vi "Receiver_Example - 2 Channel - Experiment.vi"() -> ()   [LabVIEW 2022 SP3]
panel:
  out "Iterations 2":i32
  in  "OFDM - 4QAM/16QAM":bool
  out "Error out 2":errorcluster
  in  "Tab Control 2":enum32{"OFDM - 4QAM", "16QAM"}(tab)
  in  "Tab Control":enum32{"USRP Parameters", "Rx Info", "BER"}(tab)
  in  "USRP ControledParameters":T1={"Active Antenna"="RX2", "Gain (dB)"=10.0, "Carrier Frequency"=2400000000.0, "IQ Rate"=2000000.0, "Active channels"="0"} {"IQ Rate" format="%#_6p"; "Carrier Frequency" format="%#_6p"; "Gain (dB)" format="%#_6f"}
  in  "Device selection":refnum<k15>="RIO0"
  in  "Trigger level":dbl=0.005 format="%f"
  out "?":T2
  out "SIG valid?":bool
  out "Frequency offset":dbl
  out "Coerced Parameters":T3={"IQ Rate"=100000.0, "Carrier  Freq."=100000.0, "Gain"=0.0} {"Gain" format="%#_6f"; "Carrier  Freq." format="%#_6p"; "IQ Rate" format="%#_6p"}
  out "Error out":errorcluster
  in  "Boolean":bool
  in  "Expected message LP":string="Non Critical Data\nNon Critical Data\nNon Critical Data\nNon Critical Data\nNon Critical Data"
  in  "Record BER":bool
  in  "Refresh Button":bool
  out "Inst. BER LP":dbl format="%#_4g"
  out "No. Bits LP":dbl
  out "Acum. Err LP":dbl
  out "Acc. BER LP":dbl format="%#_4g"
  in  "Expected message 2 HP":string="Critical Dataaaaa\nCritical Dataaaaa\nCritical Dataaaaa\nCritical Dataaaaa\nCritical Dataaaaa"
  out "Inst. BER HP":dbl format="%#_4g"
  out "Acum. Err HP":dbl
  out "No. Bits HP":dbl
  out "Acc. BER  HP":dbl format="%#_4g"
  out "Expected message LP Detected":string="Non Critical Data\nNon Critical Data\nNon Critical Data\nNon Critical Data\nNon Critical Data"
  out "Expected message  HP  Detected":string="Critical Dataaaaa\nCritical Dataaaaa\nCritical Dataaaaa\nCritical Dataaaaa\nCritical Dataaaaa"
  in  "Boolean 2":bool
  out "Constellation Map":cdb[](graph)
  out "Low-Power Decoded Message":string
  out "High-Power Decoded Message":string
  out "Low-Power BER Graph":dbl(graph)
  out "High-Power BER Graph":dbl(graph)
  out "Low-Power Instantaneous BER Graph":u8(slide) scale=0.0..100.0
  out "High-Power Instantaneous BER Graph":u8(slide) scale=0.0..100.0
  in  "Low-Power Window Size":dbl=15.0 format="%#_6p"
  in  "High-Power Window Size":dbl=15.0 format="%#_6p"
  out "Reconstructed Image":T4(plugin-control)
  out "Expected message  HP  Detected 2":string="Critical Dataaaaa\nCritical Dataaaaa\nCritical Dataaaaa\nCritical Dataaaaa\nCritical Dataaaaa"
  in  "Boolean 3":bool
  in  "High-Power Window Size 2":dbl=15.0 format="%#_6p"
  out "High-Power Instantaneous BER Graph 2":u8(slide) scale=0.0..100.0
  out "High-Power BER Graph 2":dbl(graph)
  out "No. Bits HP 2":dbl
  out "Acc. BER  HP 2":dbl format="%#_4g"
  out "Acum. Err HP 2":dbl
  out "Inst. BER HP 2":dbl format="%#_4g"
  in  "Expected message 2 HP 2":string="Critical Dataaaaa\nCritical Dataaaaa\nCritical Dataaaaa\nCritical Dataaaaa\nCritical Dataaaaa"
  out "High-Power Decoded Message 2":string
  in  "Record BER 2":bool
  out "Constellation Map 2":cdb[](graph)
  out "Frequency offset 2":dbl
  out "SIG valid? 2":bool
  in  "Refresh Button 2":bool
  out "Reconstructed Image":T4(plugin-control)
  out "Iterations":i32
  in  "error in (no error)":errorcluster
  # "OFDM Superposition Coded Receiver"
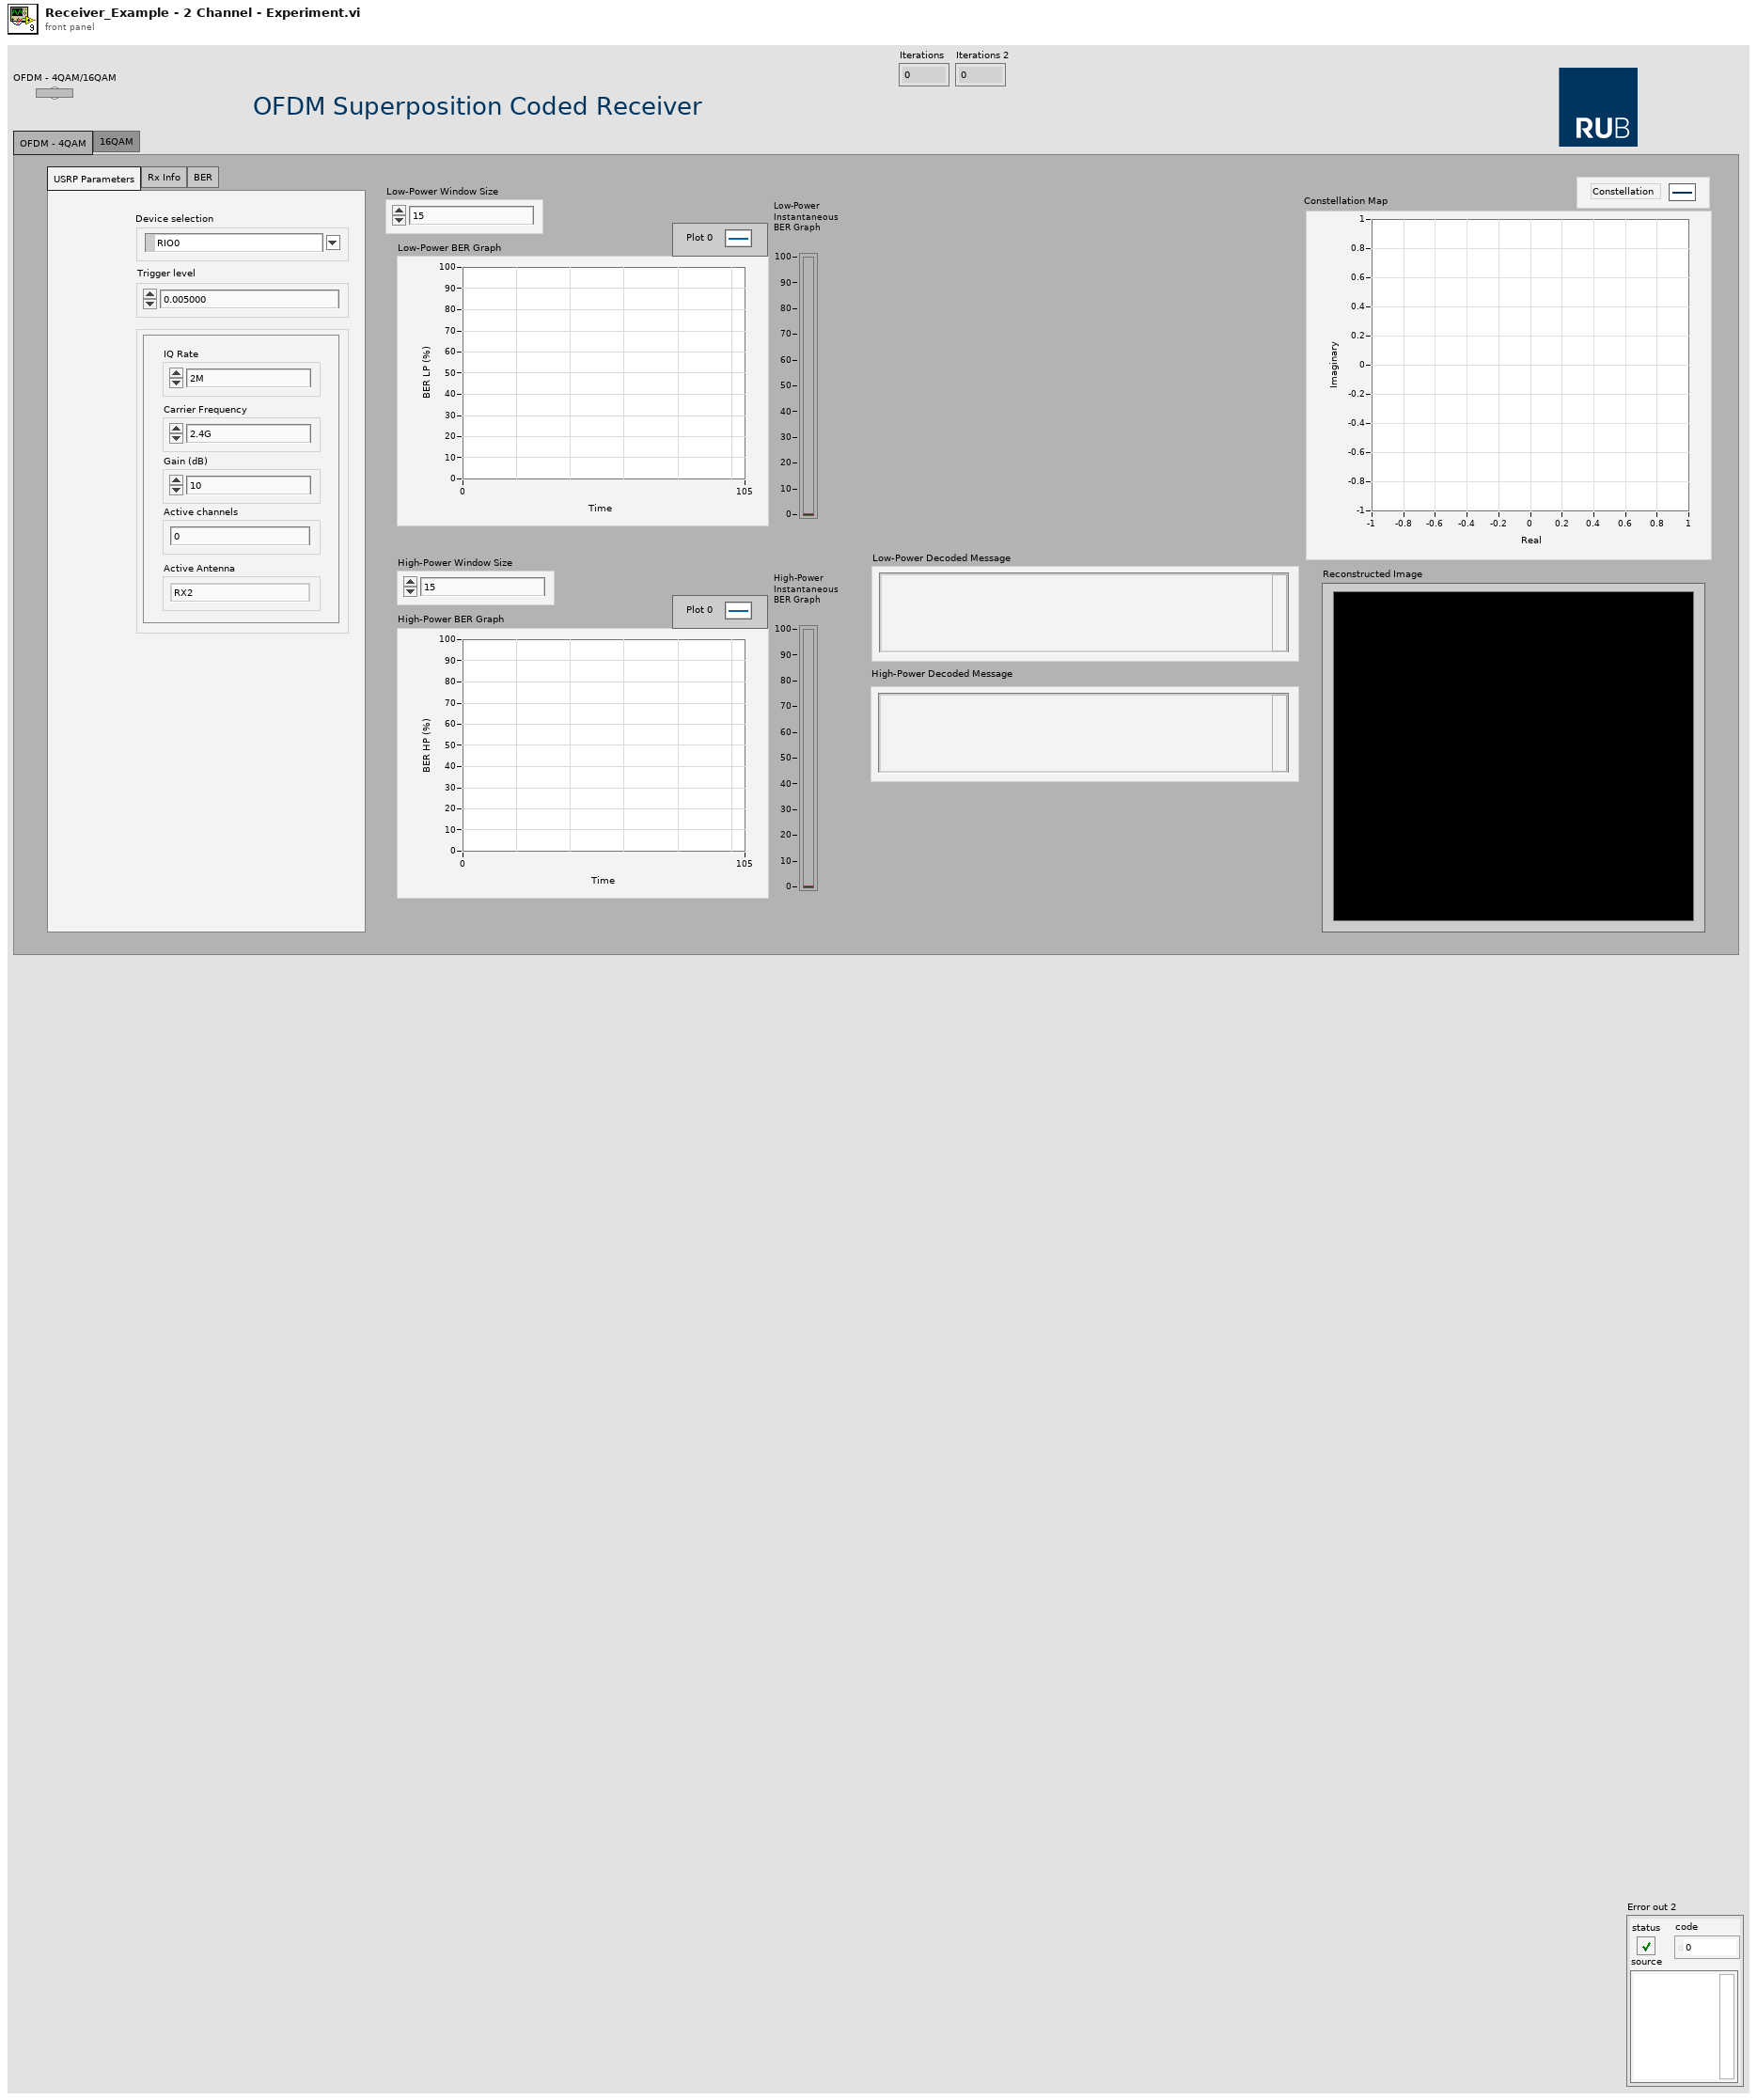
[diagram p1: front panel]
types:
  T1 = cluster{"Active Antenna":string, "Gain (dB)":dbl, "Carrier Frequency":dbl, "IQ Rate":dbl, "Active channels":string}
  T2 = cluster{"Modulation type":enum16{"QPSK(4QAM)", "64QAM", "16QAM", "BPSK"}, "BCC rate (k/n)":enum16{"1/2", "2/3", "3/4"}}
  T3 = cluster{"IQ Rate":dbl, "Carrier  Freq.":dbl, "Gain":dbl}
  T4 = typedef "IMAQ Image.ctl" = refnum<image>
  T5 = cluster{"coerced IQ rate":dbl, "coerced carrier frequency":dbl, "coerced gain":dbl}
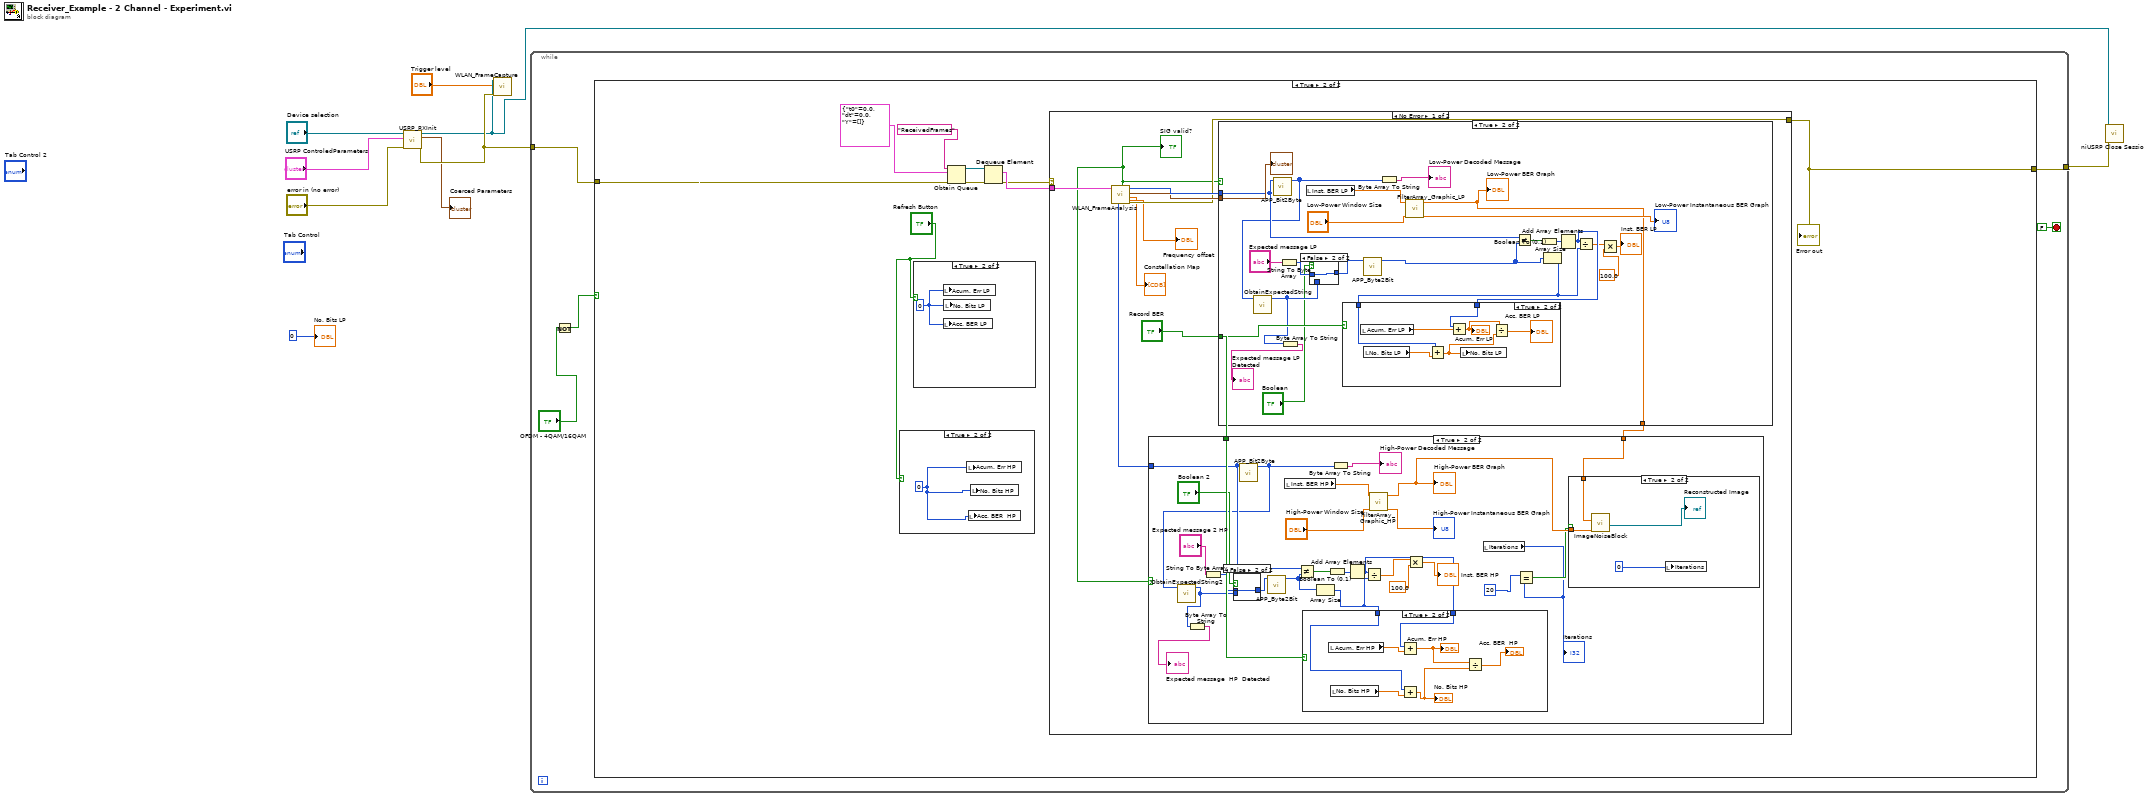
[diagram p0: block diagram]
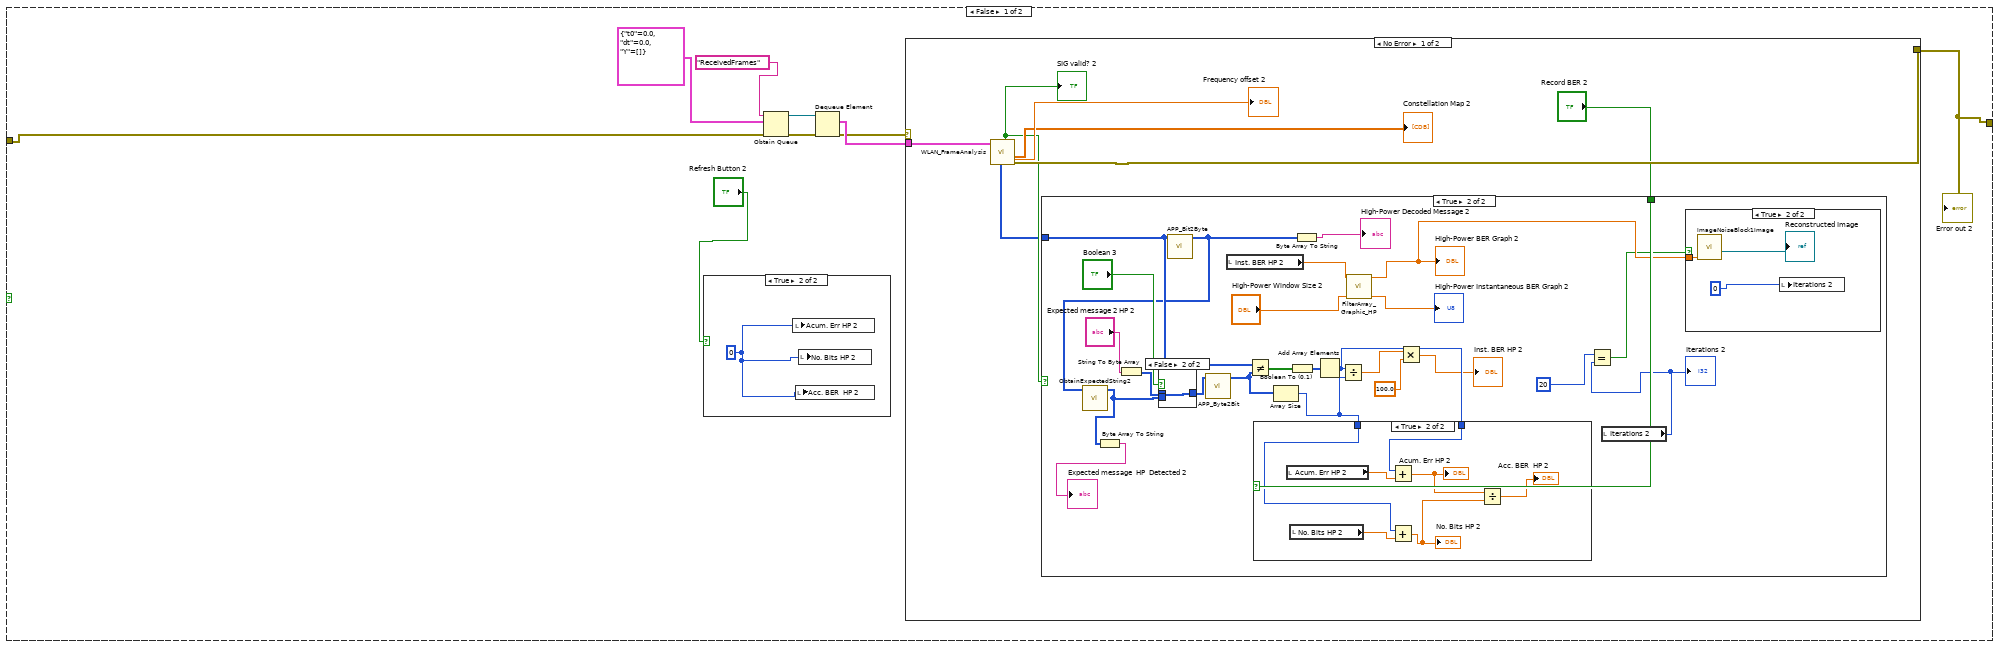
[diagram p2: hidden frame]
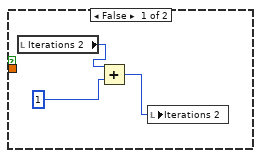
[diagram p5: hidden frame]
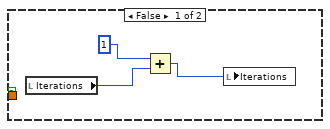
[diagram p13: hidden frame]
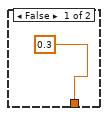
[diagram p15: hidden frame]
diagram:
  n1 = call "USRP_RXInit.vi"("device names"="Device selection", "USRP ControledParameters"="USRP ControledParameters", "error in (no error)"="error in (no error)") -> ("session handle out"=w6:refnum<k15>, "USRP CoercedParamters"=→"Coerced Parameters":T5, "error out"=w8:errorcluster)  [unwired: 5 in]
  n2 = call "WLAN_FrameCapture.vi"("error in (no error)"=w8, "Trigger level"="Trigger level", "session handle"=w6) -> ()  [unwired: 8 in]
  n3 = while {
    tunnel: w8 -> [w14]
    tunnel: [w13] -> w7
    stop <- FALSE stop-if-true
    n4 = Not(x="OFDM - 4QAM/16QAM") -> (.not. x?=w10:bool)
    n5 = case shown="True" w10 {
      tunnel: w14 -> [w16 w74]
      tunnel: [w15 w73] -> w13
      frame False {
        n6 = case shown="True" "Refresh Button 2" {
          frame False {
          }
          frame True {
            w24 = 0
            n7 = local write "Acum. Err HP 2"(w24) -> ()
            n8 = local write "Acc. BER  HP 2"(w24) -> ()
            n9 = local write "No. Bits HP 2"(w24) -> ()
          }
        }
        n10 = Obtain Queue(name (unnamed)="ReceivedFrames", element data type=cluster{"t0":dbl, "dt":dbl, "Y":cdb[]} {"t0"=0.0, "dt"=0.0, "Y"=[]} ("data"), error in (no error)=w16) -> (queue out=w17:refnum<queue>, error out=w20:errorcluster)  [unwired: 2 in, 1 out]
        n11 = Dequeue Element(queue=w17, error in (no error)=w20) -> (element=w19:cluster{"t0":dbl, "dt":dbl, "Y":cdb[]}, error out=w18:errorcluster)  [unwired: 1 in, 2 out]
        n12 = case shown="No Error" w18 {
          selector: w18 -> [_ w72]
          tunnel: w19 -> [w30 _]
          tunnel: [w31 w72] -> w15
          frame No Error {
            n13 = call "WLAN_FrameAnalysis.vi"("input cluster"=w30) -> ("error out"=w31:errorcluster, "Constellation"=→"Constellation Map 2":cdb[], "Frequency offset"=→"Frequency offset 2":dbl, "SIG valid?"=w26:bool, "outputbitsHP"=w25:i8[])  [unwired: 4 in, 2 out]
            "SIG valid? 2" <- w26
            n14 = case shown="True" w26 {
              tunnel: "Record BER 2" -> [_ w50]
              tunnel: w25 -> [_ w45]
              frame False {
              }
              frame True {
                n15 = String To Byte Array(string="Expected message 2 HP 2") -> (unsigned byte array=w43:u8[])
                n16 = call "APP_Bit2Byte.vi"("input bit stream"=w45) -> ("output byte stream"=w39:u8[])  [unwired: 10 in]
                n17 = call "ObtainExpectedString2.vi"("Array"=w39) -> ("detectedMessage"=w41:i8[])  [unwired: 9 in]
                n18 = Byte Array To String(unsigned byte array=w41) -> (string=→"Expected message  HP  Detected 2":string)
                n19 = case shown="False" "Boolean 3" {
                  tunnel: [w63 w64] -> w44
                  tunnel: w43 -> [_ w64]
                  tunnel: w41 -> [w63 _]
                  frame True {
                  }
                  frame False {
                  }
                }
                n20 = call "APP_Byte2Bit.vi"("input byte stream"=w44) -> ("output bit stream"=w46:i8[])  [unwired: 10 in]
                n21 = local read "Inst. BER HP 2"() -> (w49:dbl)
                n22 = Not Equal?(x=w45, y=w46) -> (x != y?=w54:bool[])
                n23 = Array Size(array=w46) -> (size(s)=w51:i32)
                n24 = Boolean To (0,1)(Boolean=w54) -> (0, 1=w53:i16[])
                n25 = Byte Array To String(unsigned byte array=w39) -> (string=→"High-Power Decoded Message 2":string)
                n26 = Add Array Elements(numeric array=w53) -> (sum=w52:i16)
                n27 = case shown="True" w50 {
                  tunnel: w52 -> [_ w70]
                  tunnel: w51 -> [_ w65]
                  frame False {
                  }
                  frame True {
                    n28 = local read "Acum. Err HP 2"() -> (w71:dbl)
                    n29 = local read "No. Bits HP 2"() -> (w67:dbl)
                    n30 = Add(x=w70, y=w71) -> (x+y=w69:dbl)
                    "Acum. Err HP 2" <- w69
                    n31 = Add(x=w65, y=w67) -> (x+y=w66:dbl)
                    "No. Bits HP 2" <- w66
                    n32 = Divide(x=w69, y=w66) -> (x/y=→"Acc. BER  HP 2":dbl)
                  }
                }
                n33 = Divide(x=w52, y=w51) -> (x/y=w38:dbl)
                n34 = call "FilterArray_Graphic_HP.vi"("Window Size"="High-Power Window Size 2", "Instantaneous BER"=w49) -> ("Slide Bar"=→"High-Power Instantaneous BER Graph 2":dbl, "Graph Instantaneous BER"=w35:dbl)  [unwired: 4 in]
                "High-Power BER Graph 2" <- w35
                n35 = Multiply(x=w38, y=100.0) -> (x*y=→"Inst. BER HP 2":dbl)
                n36 = local read "Iterations 2"() -> (w33:i32)
                "Iterations 2" <- w33
                n37 = Equal?(x=20, y=w33) -> (x = y?=w32:bool)
                n38 = case shown="True" w32 {
                  tunnel: w35 -> [_ w62]
                  frame False {
                    n39 = local read "Iterations 2"() -> (w59:i32)
                    n40 = Add(x=w59, y=1) -> (x+y=w57:i32)
                    n41 = local write "Iterations 2"(w57) -> ()
                  }
                  frame True {
                    n42 = call "ImageNoiseBlock1Image.vi"("BERHP"=w62) -> ("High-Power Image"=→"Reconstructed Image":T4)  [unwired: 9 in]
                    n43 = local write "Iterations 2"(0) -> ()
                  }
                }
              }
            }
          }
          frame Error {
          }
        }
        "Error out 2" <- w15
      }
      frame True {
        n44 = case shown="True" "Refresh Button" {
          frame False {
          }
          frame True {
            w82 = 0
            n45 = local write "Acum. Err HP"(w82) -> ()
            n46 = local write "Acc. BER  HP"(w82) -> ()
            n47 = local write "No. Bits HP"(w82) -> ()
          }
        }
        n48 = case shown="True" "Refresh Button" {
          frame False {
          }
          frame True {
            w83 = 0
            n49 = local write "Acum. Err LP"(w83) -> ()
            n50 = local write "Acc. BER LP"(w83) -> ()
            n51 = local write "No. Bits LP"(w83) -> ()
          }
        }
        n52 = Obtain Queue(name (unnamed)="ReceivedFrames", element data type=cluster{"t0":dbl, "dt":dbl, "Y":cdb[]} {"t0"=0.0, "dt"=0.0, "Y"=[]} ("data"), error in (no error)=w74) -> (queue out=w75:refnum<queue>, error out=w78:errorcluster)  [unwired: 2 in, 1 out]
        n53 = Dequeue Element(queue=w75, error in (no error)=w78) -> (element=w77:cluster{"t0":dbl, "dt":dbl, "Y":cdb[]}, error out=w76:errorcluster)  [unwired: 1 in, 2 out]
        n54 = case shown="No Error" w76 {
          selector: w76 -> [_ w169]
          tunnel: w77 -> [w90 _]
          tunnel: [w91 w169] -> w73
          frame No Error {
            n55 = call "WLAN_FrameAnalysis.vi"("input cluster"=w90) -> ("error out"=w91:errorcluster, "Constellation"=→"Constellation Map":cdb[], "Modulation parameter"=w92:T2, "output bits"=w93:i8[], "Frequency offset"=→"Frequency offset":dbl, "SIG valid?"=w86:bool, "outputbitsHP"=w85:i8[])  [unwired: 4 in]
            "SIG valid?" <- w86
            n56 = case shown="True" w86 {
              tunnel: w93 -> [_ w144]
              tunnel: w92 -> [_ w159]
              tunnel: "Record BER" -> [_ w153]
              tunnel: [0.3 ("Graph Instantaneous BER") w149] -> w84
              frame False {
              }
              frame True {
                n57 = call "APP_Bit2Byte.vi"("input bit stream"=w144) -> ("output byte stream"=w140:u8[])  [unwired: 10 in]
                n58 = call "ObtainExpectedString.vi"("Array"=w140) -> ("detectedMessage"=w142:i8[])  [unwired: 9 in]
                n59 = String To Byte Array(string="Expected message LP") -> (unsigned byte array=w145:u8[])
                n60 = Byte Array To String(unsigned byte array=w142) -> (string=→"Expected message LP Detected":string)
                n61 = local read "Inst. BER LP"() -> (w152:dbl)
                n62 = case shown="False" "Boolean" {
                  tunnel: [w160 w161] -> w146
                  tunnel: w145 -> [_ w161]
                  tunnel: w142 -> [w160 _]
                  frame True {
                  }
                  frame False {
                  }
                }
                n63 = call "APP_Byte2Bit.vi"("input byte stream"=w146) -> ("output bit stream"=w147:i8[])  [unwired: 10 in]
                n64 = Byte Array To String(unsigned byte array=w140) -> (string=→"Low-Power Decoded Message":string)
                n65 = call "FilterArray_Graphic_LP.vi"("Window Size"="Low-Power Window Size", "Instantaneous BER"=w152) -> ("Slide Bar"=→"Low-Power Instantaneous BER Graph":dbl, "Graph Instantaneous BER"=w149:dbl)  [unwired: 4 in]
                "Low-Power BER Graph" <- w149
                n66 = Not Equal?(x=w144, y=w147) -> (x != y?=w155:bool[])
                n67 = Boolean To (0,1)(Boolean=w155) -> (0, 1=w148:i16[])
                n68 = Array Size(array=w147) -> (size(s)=w157:i32)
                n69 = Add Array Elements(numeric array=w148) -> (sum=w154:i16)
                n70 = case shown="True" w153 {
                  tunnel: w157 -> [_ w167]
                  tunnel: w154 -> [_ w165]
                  frame False {
                  }
                  frame True {
                    n71 = local read "Acum. Err LP"() -> (w166:dbl)
                    n72 = local read "No. Bits LP"() -> (w168:dbl)
                    n73 = Add(x=w167, y=w168) -> (x+y=w162:dbl)
                    n74 = Add(x=w165, y=w166) -> (x+y=w164:dbl)
                    "Acum. Err LP" <- w164
                    n75 = local write "No. Bits LP"(w162) -> ()
                    n76 = Divide(x=w164, y=w162) -> (x/y=→"Acc. BER LP":dbl)
                  }
                }
                n77 = Divide(x=w154, y=w157) -> (x/y=w139:dbl)
                n78 = Multiply(x=w139, y=100.0) -> (x*y=→"Inst. BER LP":dbl)
                "?" <- w159
              }
            }
            n79 = case shown="True" w86 {
              tunnel: "Record BER" -> [_ w113]
              tunnel: w85 -> [_ w103]
              tunnel: w84 -> [_ w108]
              frame False {
              }
              frame True {
                n80 = String To Byte Array(string="Expected message 2 HP") -> (unsigned byte array=w101:u8[])
                n81 = call "APP_Bit2Byte.vi"("input bit stream"=w103) -> ("output byte stream"=w97:u8[])  [unwired: 10 in]
                n82 = call "ObtainExpectedString2.vi"("Array"=w97) -> ("detectedMessage"=w99:i8[])  [unwired: 9 in]
                n83 = Byte Array To String(unsigned byte array=w99) -> (string=→"Expected message  HP  Detected":string)
                n84 = case shown="False" "Boolean 2" {
                  tunnel: [w120 w121] -> w102
                  tunnel: w101 -> [_ w121]
                  tunnel: w99 -> [w120 _]
                  frame True {
                  }
                  frame False {
                  }
                }
                n85 = call "APP_Byte2Bit.vi"("input byte stream"=w102) -> ("output bit stream"=w107:i8[])  [unwired: 10 in]
                n86 = local read "Inst. BER HP"() -> (w112:dbl)
                n87 = Not Equal?(x=w103, y=w107) -> (x != y?=w117:bool[])
                n88 = Array Size(array=w107) -> (size(s)=w114:i32)
                n89 = Boolean To (0,1)(Boolean=w117) -> (0, 1=w116:i16[])
                n90 = Byte Array To String(unsigned byte array=w97) -> (string=→"High-Power Decoded Message":string)
                n91 = Add Array Elements(numeric array=w116) -> (sum=w115:i16)
                n92 = case shown="True" w113 {
                  tunnel: w115 -> [_ w134]
                  tunnel: w114 -> [_ w129]
                  frame False {
                  }
                  frame True {
                    n93 = local read "Acum. Err HP"() -> (w135:dbl)
                    n94 = local read "No. Bits HP"() -> (w131:dbl)
                    n95 = Add(x=w134, y=w135) -> (x+y=w133:dbl)
                    "Acum. Err HP" <- w133
                    n96 = Add(x=w129, y=w131) -> (x+y=w130:dbl)
                    "No. Bits HP" <- w130
                    n97 = Divide(x=w133, y=w130) -> (x/y=→"Acc. BER  HP":dbl)
                  }
                }
                n98 = Divide(x=w115, y=w114) -> (x/y=w96:dbl)
                n99 = call "FilterArray_Graphic_HP.vi"("Window Size"="High-Power Window Size", "Instantaneous BER"=w112) -> ("Slide Bar"=→"High-Power Instantaneous BER Graph":dbl, "Graph Instantaneous BER"=w109:dbl)  [unwired: 4 in]
                "High-Power BER Graph" <- w109
                n100 = Multiply(x=w96, y=100.0) -> (x*y=→"Inst. BER HP":dbl)
                n101 = local read "Iterations"() -> (w105:i32)
                "Iterations" <- w105
                n102 = Equal?(x=20, y=w105) -> (x = y?=w106:bool)
                n103 = case shown="True" w106 {
                  tunnel: w109 -> [_ w128]
                  tunnel: w108 -> [_ w127]
                  frame False {
                    n104 = local read "Iterations"() -> (w122:i32)
                    n105 = Add(x=1, y=w122) -> (x+y=w123:i32)
                    n106 = local write "Iterations"(w123) -> ()
                  }
                  frame True {
                    n107 = call "ImageNoiseBlock.vi"("BERLP"=w127, "BERHP"=w128) -> ("High-Power Image"=→"Reconstructed Image":T4)  [unwired: 8 in]
                    n108 = local write "Iterations"(0) -> ()
                  }
                }
              }
            }
          }
          frame Error {
          }
        }
        "Error out" <- w73
      }
    }
  }
  n109 = call <instrlib>:"niUSRP Close Session.vi"("session handle"=w6, "error in (no error)"=w7) -> ()  [unwired: 13 in, 1 out]
  "No. Bits LP" <- 0
